vi "Simple Smith Plot.vi"() -> ()   [LabVIEW 2023]
doc: "Uses the Smith Plot VI to draw a smith plot in a picture indicator. This example shows how the Smith Plot VIs autoscale the displayed data."
panel:
  in  "Stop":bool
  in  "Autoscale":bool=TRUE
  out "Smith Plot":picture
  # "Overview: Uses the Smith Plot VI to draw a smith plot in a picture indicator.\nInstructions:\n1. Run the VI.\n2. Toggle the Autoscale control to view the plot with autoscaling on or off.\n3. Click Stop to stop the VI."
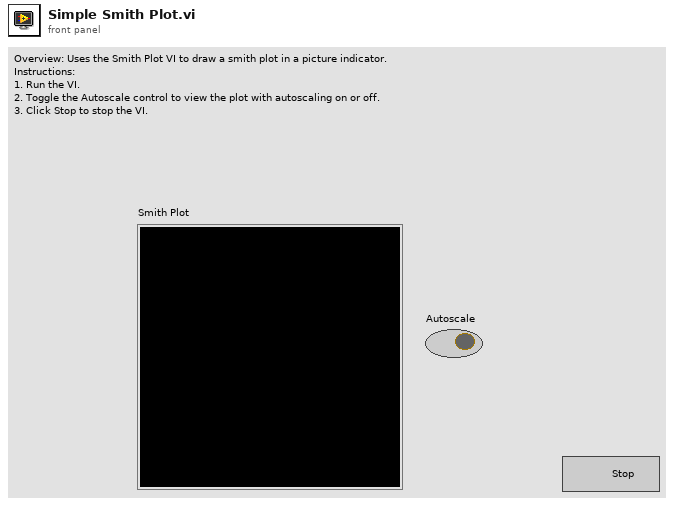
[diagram p1: front panel]
types:
  T1 = cluster{"x minimum":dbl, "x maximum":dbl, "y minimum":dbl, "y maximum":dbl}
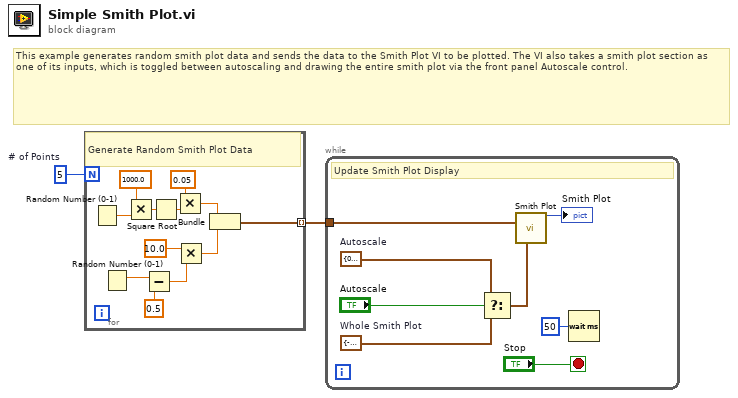
[diagram p0: block diagram]
diagram:
  w2 = 5  # # of Points
  # "This example generates random smith plot data and sends the data to the Smith Plot VI to be plotted. The VI also takes a smith plot section as one of its inputs, which is toggled between autoscaling and drawing the entire smith plot via the front panel Autoscale control."
  n1 = for {
    N: w2 -> [_]
    tunnel: [w8] -> w1 mode=indexing
    # "Generate Random Smith Plot Data"
    n2 = Random Number (0-1)() -> (number: 0 to 1=w14:dbl)
    n3 = Random Number (0-1)() -> (number: 0 to 1=w11:dbl)
    n4 = Multiply(x=1000.0, y=w14) -> (x*y=w10:dbl)
    n5 = Subtract(x=w11, y=0.5) -> (x-y=w12:dbl)
    n6 = Square Root(x=w10) -> (sqrt(x)=w7:dbl)
    n7 = Multiply(x=0.05, y=w7) -> (x*y=w6:dbl)
    n8 = Multiply(x=10.0, y=w12) -> (x*y=w9:dbl)
    n9 = Bundle(w6, w9) -> (w8:cluster{dbl, dbl})  [unwired: 1 in]
  }
  n10 = while {
    tunnel: w1 -> [w16]
    stop <- "Stop" stop-if-true
    w20 = T1 {"x minimum"=0.0, "x maximum"=0.0, "y minimum"=0.0, "y maximum"=0.0}  # Autoscale
    w22 = T1 {"x minimum"=-1.0, "x maximum"=1.0, "y minimum"=-1.0, "y maximum"=1.0}  # Whole Smith Plot
    # "Update Smith Plot Display"
    n11 = Select(t=w20, s="Autoscale", f=w22) -> (s? t:f=w18:T1)
    n12 = call <vilib>:"Smith Plot.vi"("smith plot"=w16, "smith plot section"=w18) -> ("new picture"=→"Smith Plot":picture)  [unwired: 13 in]
    n13 = Wait (ms)(milliseconds to wait=u32 50) -> ()  [unwired: 1 out]
  }
